vi "Test Read State File.vi"() -> ()   [LabVIEW 2013]
doc: "This VI tests whether we can read states from our provided colon-delimited state file."
panel:
  out "State List":dbl[][](array[numeric])
  in  "file path (use dialog)":path=path "C:/Users/Nathan/Documents/LV_testRig-Dev/Data/state_sequence.txt"
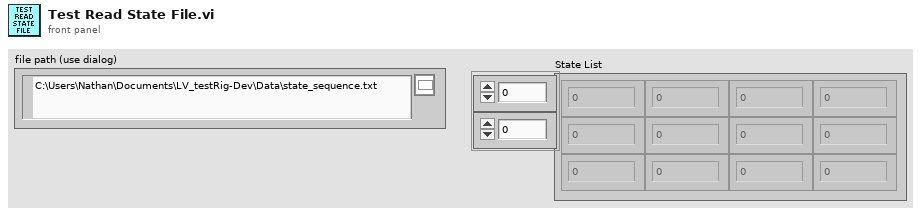
[diagram p1: front panel]
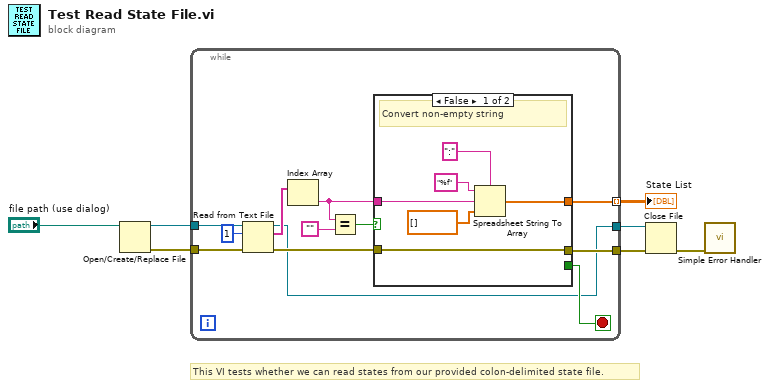
[diagram p0: block diagram]
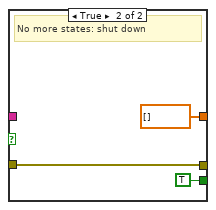
[diagram p2: hidden frame]
diagram:
  # "This VI tests whether we can read states from our provided colon-delimited state file."
  n1 = Open/Create/Replace File(file path (use dialog)="file path (use dialog)") -> (refnum out=w6:refnum<file>, error out=w5:errorcluster)  [unwired: 5 in, 1 out]
  n2 = while {
    tunnel: w6 -> [w19]
    tunnel: w5 -> [w18]
    tunnel: [w11] -> w3
    tunnel: [w9] -> w4 mode=indexing
    tunnel: [w8] -> w2
    stop <- w10 stop-if-true
    n3 = Read from Text File(file (use dialog)=w19, count=1, error in=w18) -> (refnum out=w8:refnum<file>, text=w14:string[], error out=w13:errorcluster)  [unwired: 1 in, 1 out]
    n4 = Index Array(array=w14) -> (element=w12:string)  [unwired: 1 in]
    n5 = Equal?(x=w12, y="") -> (x = y?=w15:bool)
    n6 = case shown="False" w15 {
      tunnel: [w22 dbl[] []] -> w9
      tunnel: w13 -> [w20 w27]
      tunnel: w12 -> [w21 _]
      tunnel: [w20 w27] -> w11
      tunnel: [_ TRUE] -> w10
      frame False {
        # "Convert non-empty string"
        n7 = Spreadsheet String To Array(delimiter (Tab)=":", format string="%f", spreadsheet string=w21, array type (2D Dbl)=dbl[] []) -> (array=w22:dbl[])
      }
      frame True {
        # "No more states: shut down"
      }
    }
  }
  "State List" <- w4
  n8 = Close File(refnum=w2, error in=w3) -> (error out=w1:errorcluster)  [unwired: 1 out]
  n9 = call <vilib>:"Simple Error Handler.vi"("error in (no error)"=w1) -> ()  [unwired: 4 in, 5 out]
